vi "Read Base path.vi"(8 "error in (no error)":errorcluster, 11 "SC-Main in":refnum<class "HC-Main.lvclass">) -> (0 "error out":errorcluster, 2 "Base path":path, 3 "SC-Main out":refnum<class "HC-Main.lvclass">)   [LabVIEW 2013, in "HardwareCharacterization.lvlib" / "HC-Main.lvclass"]
uses:
  HC-Main.lvclass
  HC-Main.lvclass/HC-Main.ctl
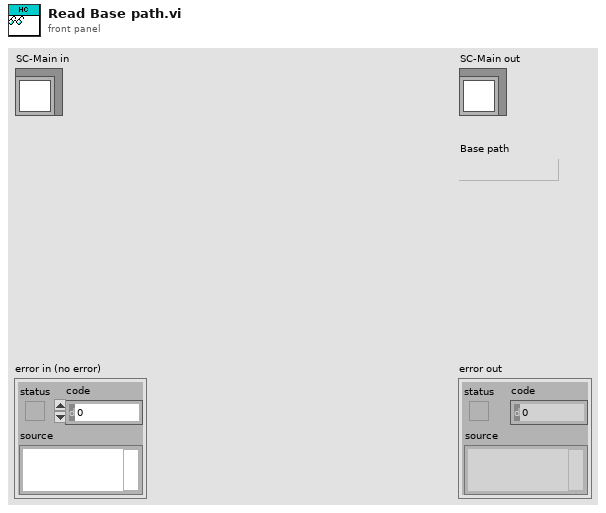
[diagram p1: front panel]
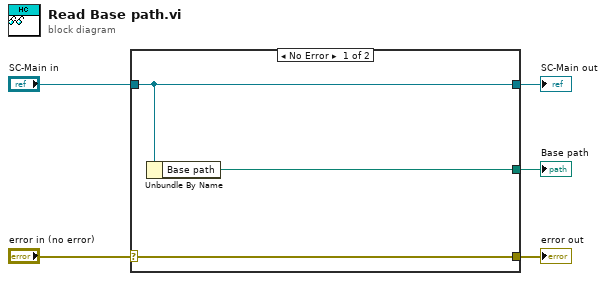
[diagram p0: block diagram]
diagram:
  n1 = case shown="No Error" "error in (no error)" {
    selector: "error in (no error)" -> [w8 w9]
    tunnel: [w8 w9] -> w4
    tunnel: [w7 w10] -> w2
    tunnel: "SC-Main in" -> [w7 w10]
    tunnel: [w6 _] -> w1
    frame No Error {
      n2 = Unbundle By Name(w7) -> ("Base path"=w6:path)
    }
    frame Error {
    }
  }
  "error out" <- w4
  "SC-Main out" <- w2
  "Base path" <- w1
